vi "Initialize.vi"(7 "Channel Name":string="ActualValue.ch%d.AV", 8 "error in":errorcluster, 9 "Number of Channels":u32=1, 10 "Instance Name":string, 11 "Actual Value in":refnum<class "Actual Value.lvclass">) -> (0 "error out":errorcluster, 2 "Channel":T1[](array[typedef]), 3 "Actual Value out":refnum<class "Actual Value.lvclass">)   [LabVIEW 2023, in "Actual Value.lvclass"]
uses:
  Actual Value.lvclass
  Utilities/Channel.ctl
  Actual Value.lvclass/Actual Value.ctl
  <vilib>/ADAS Replay HIL/Channels/Tag Wrapper/Polymorphic/Open Producer Tag (Double).vi
  <vilib>/ADAS Replay HIL/Channels/Tag Wrapper/Polymorphic/Set Default Value (Double).vi
  <vilib>/ADAS Replay HIL/Channels/Tag Wrapper/Polymorphic/Open Producer Tag (Double).vi/45cd6eaa-a1ce-41a4-8aba-62a49d103d7e.vi
  <vilib>/ADAS Replay HIL/Channels/Tag Wrapper/Polymorphic/Set Default Value (Double).vi/228e99de-6fcf-414d-86fc-dc277c7b351f.vi
  <vilib>/ADAS Replay HIL/Channels/Tag Wrapper/Polymorphic/Open Producer Tag (Double).vi/45cd6eaa-a1ce-41a4-8aba-62a49d103d7e.vi/c28b0ead-42ad-4072-80a2-aca7f2bd7ce3.vi
  <vilib>/ADAS Replay HIL/Channels/Tag Wrapper/Polymorphic/Set Default Value (Double).vi/228e99de-6fcf-414d-86fc-dc277c7b351f.vi/4bc1c15b-36ab-481f-b8dd-c64075ce723a.vi
  <vilib>/ADAS Replay HIL/AdasHilServices/AdasHilServices Fill In Error Info Ex.vi
  <vilib>/ADAS Replay HIL/Channels/Tag Wrapper/Tag Wrapper.lvlib
  Utilities/Utilities.lvlib
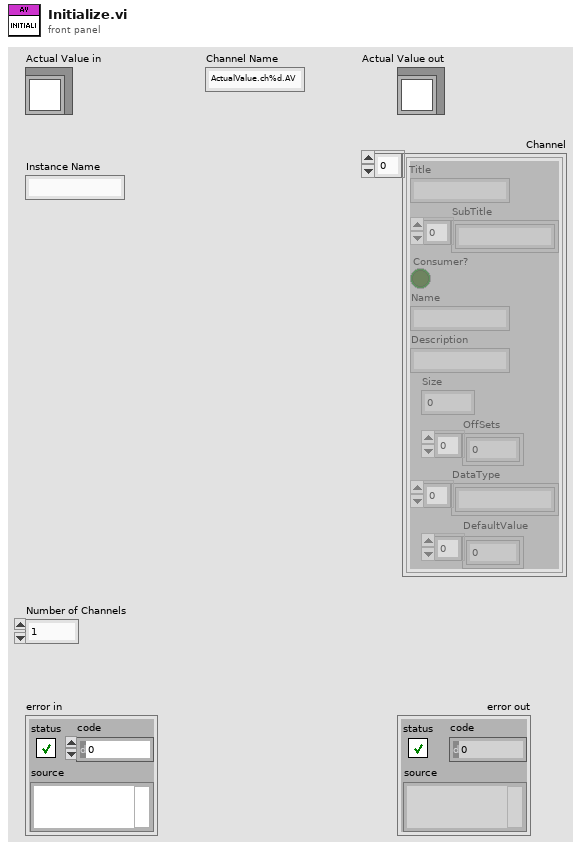
[diagram p1: front panel]
types:
  T1 = typedef "Utilities.lvlib/Channel.ctl" = cluster{"Title":string, "SubTitle":string[], "Consumer?":bool, "Name":string, "Description":string, "Size":i32, "OffSets":i32[], "DataType":string[], "DefaultValue":dbl[]}
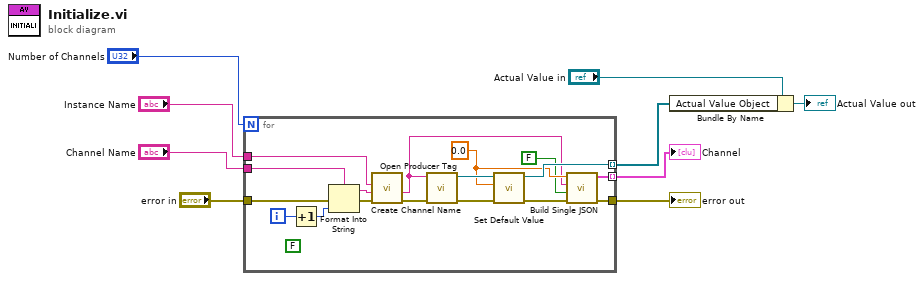
[diagram p0: block diagram]
diagram:
  n1 = for {
    N: "Number of Channels" -> [_]
    tunnel: [w21] -> w3 mode=indexing
    tunnel: [w10] -> w6
    tunnel: "Channel Name" -> [w16]
    tunnel: "Instance Name" -> [w19]
    tunnel: "error in" -> [w24]
    tunnel: [w12] -> w1 mode=indexing
    i -> [w26]
    (unwired) FALSE ("Consumer?")
    w15 = 0.0 ("Default Value")
    n2 = Increment(x=w26) -> (x+1=w25:i32)
    n3 = Format Into String(format string=w16, error in=w24, w25) -> (resulting string=w20:string, error out=w18:errorcluster)  [unwired: 1 in]
    n4 = call "Create Channel Name.vi"("error in"=w18, "Channel Name"=w20, "Plugin Name"=w19) -> ("error out"=w17:errorcluster, "Data Channel Name"=w14:string)  [unwired: 7 in]
    n5 = call-poly <vilib>:"Open Producer Tag.vi"("error in"=w17, "Channel Name"=w14) -> ("error out"=w23:errorcluster, "ADAS HIL Channel"=w22:refnum<k21>)  [unwired: 8 in]
    n6 = call-poly <vilib>:"Set Default Value.vi"("error in"=w23, "Default Value"=w15, "ADAS HIL Channel in"=w22) -> ("error out"=w11:errorcluster, "ADAS HIL Channel out"=w21:refnum<k21>)  [unwired: 7 in]
    n7 = call "Build Single JSON.vi"("error in"=w11, "Consumer?"=FALSE, "ChannelName"=w14, "Single"=w15) -> ("error out"=w10:errorcluster, "Channel"=w12:T1)  [unwired: 6 in]
  }
  "error out" <- w6
  "Channel" <- w1
  n8 = Bundle By Name(cluster="Actual Value in", "Actual Value Object"=w3) -> (→"Actual Value out":refnum<class "Actual Value.lvclass">)
